vi "Fetch Waveform (Waveform Data Type)2.vi"(8 "error in (no error)":errorcluster, 9 "Maximum Time (10000ms)":u32=10000, 10 "Channel (0: Channel 1)":u16(ring) items=["Channel 1", "Channel 2", "Channel 3", "Channel 4", "Math", "Reference 1", "Reference 2", "Reference 3", "Reference 4", "D0", "D1", "D2", "D3", "D4", "D5", "D6", "D7", "D8", "D9", "D10", "D11", "D12", "D13", "D14", "D15", "Amplitude", "Frequency", "Phase", "Normal", "Average", "Maximum Peak Hold", "Minimum Peak Hold"], 11 "VISA resource name":refnum<visa-resource-name>) -> (0 "error out":errorcluster, 2 "Waveform Data":waveform(dbl)(graph), 3 "VISA resource name out":refnum<visa-resource-name>)   [LabVIEW 2011]
doc: "Returns the waveform that an oscilloscope acquires for a channel you specify. An acquisition that you initiate before calling this VI generates the waveform.\n\nYou first enable channels with the Configure Channel VI. Then you use the Initiate VI to start an acquisition on the enabled channels. An oscilloscope concurrently acquires waveforms for these channels. You must call the Fetch Waveform VI separately to obtain waveforms for each enabled channel.\nHowever, you also can call the Read Waveform VI instead of using the above low-level VIs.\n\n<B>Note</B>: Use the Fetch Waveform VI only with other low-level VIs, such as the Initiate VI, the Abort VI, and the Fetch Waveform Measurement VI. High-level VIs, such as the Read Waveform VI, automatically incorporate the functions of the Initiate VI and the Fetch Waveform VI. The Fetch Waveform VI does not check the status of an instrument."
uses:
  <instrlib>/Tektronix DPO MSO 2000 4000 Series/Tektronix DPO MSO 2000 4000 Series.lvlib
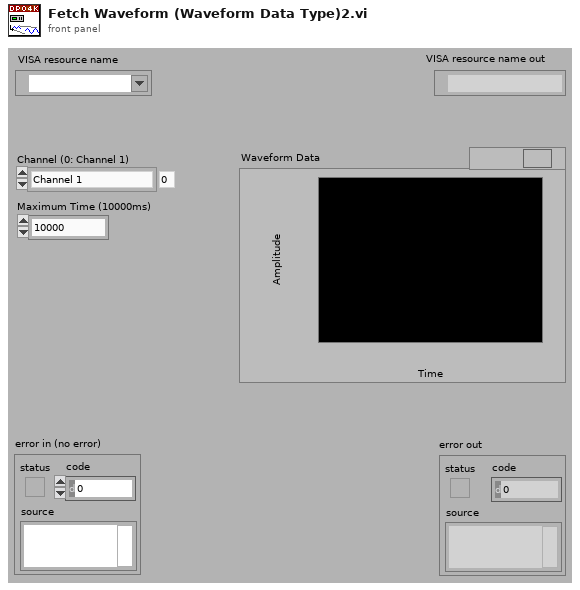
[diagram p1: front panel]
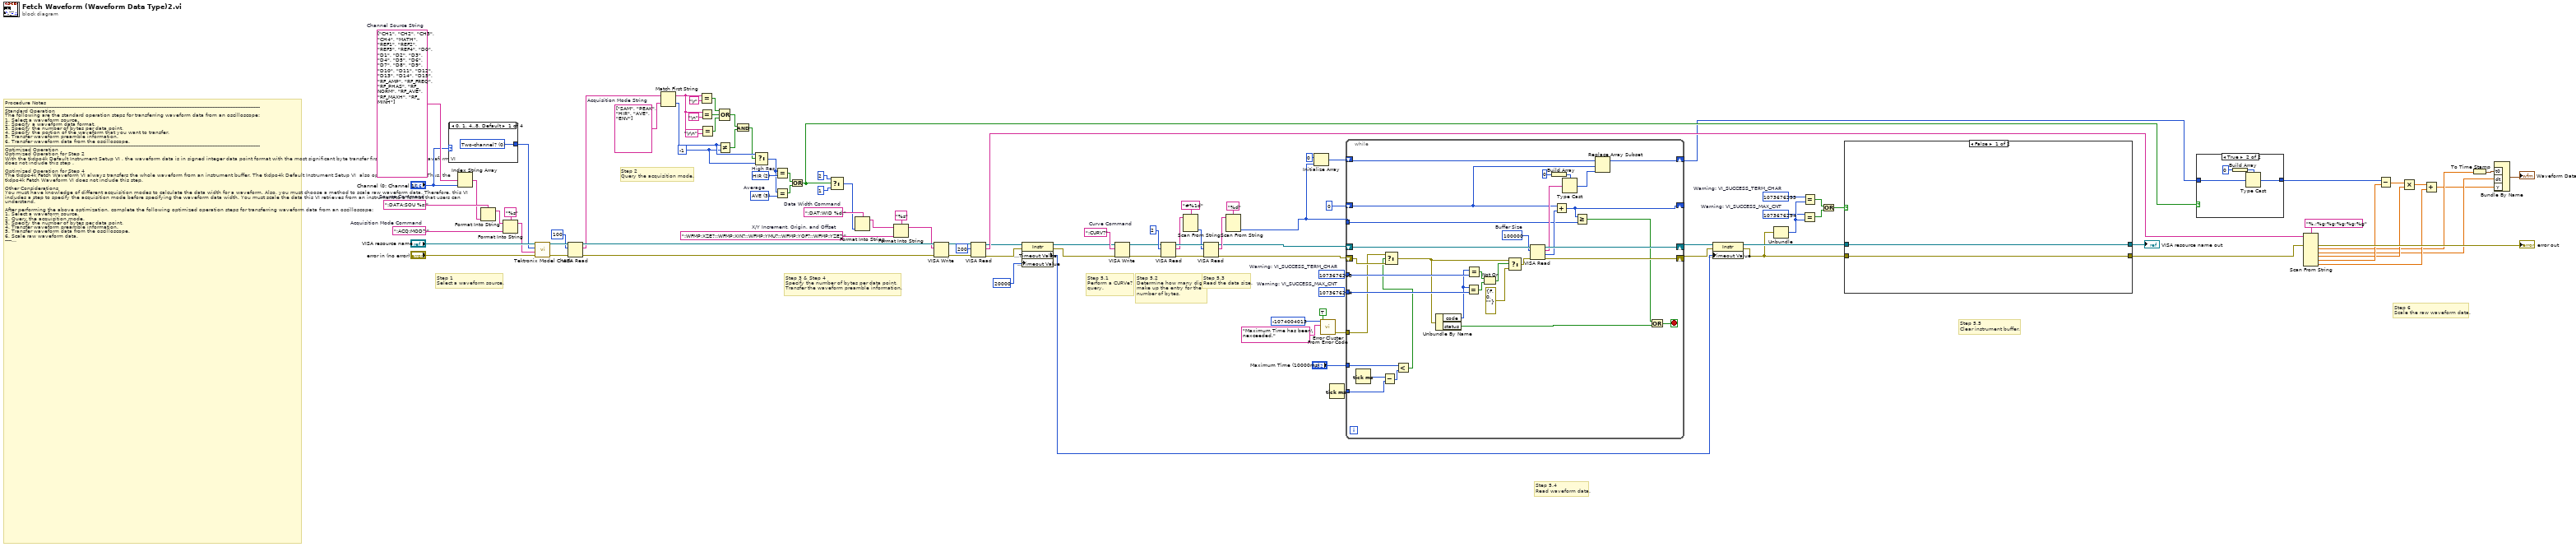
[diagram p0: block diagram]
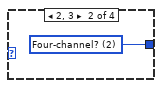
[diagram p2: hidden frame]
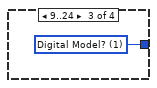
[diagram p3: hidden frame]
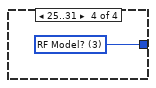
[diagram p4: hidden frame]
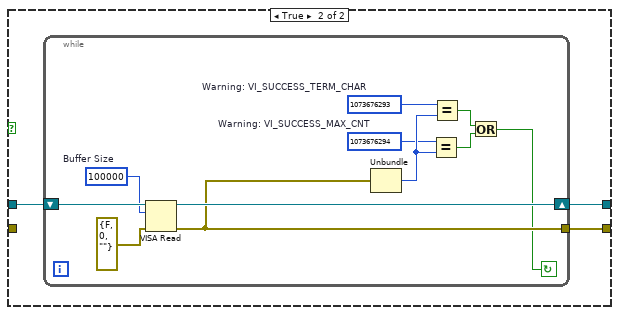
[diagram p6: hidden frame]
diagram:
  w44 = 1073676294  # Warning: VI_SUCCESS_MAX_CNT
  w45 = 1073676293  # Warning: VI_SUCCESS_TERM_CHAR
  w48 = 1073676294  # Warning: VI_SUCCESS_MAX_CNT
  w47 = 1073676293  # Warning: VI_SUCCESS_TERM_CHAR
  w57 = -1 ("y")
  w84 = ":CURV?"  # Curve Command
  w94 = ":DAT:WID %d;"  # Data Width Command
  w99 = u16 3 items=["SAM", "PEAK", "HIR", "AVE", "ENV"]  # Average
  w100 = u16 2 items=["SAM", "PEAK", "HIR", "AVE", "ENV"]  # High Res
  w69 = string[] ["SAM", "PEAK", "HIR", "AVE", "ENV"]  # Acquisition Mode String
  w93 = ":ACQ:MOD?;"  # Acquisition Mode Command
  w105 = string[] ["CH1", "CH2", "CH3", "CH4", "MATH", "REF1", "REF2", "REF3", "REF4", "D0", "D1", "D2", "D3", "D4", "D5", "D6", "D7", "D8", "D9", "D10", "D11", "D12", "D13", "D14", "D15", "RF_AMP", "RF_FREQ", "RF_PHAS", "RF_NORM", "RF_AVE", "RF_MAXH", "RF_MINH"]  # Channel Source String
  w104 = ":DATA:SOU %s;"  # Source Command
  w91 = ":WFMP:XZE?;:WFMP:XIN?;:WFMP:YMU?;:WFMP:YOF?;:WFMP:YZE?;"  # X/Y Increment, Origin, and Offset
  # "Step 6    \nScale the raw waveform data."
  # "Step 5.5    \nClear instrument buffer."
  # "Step 5.4   \nRead waveform data."
  # "Step 5.3      \nRead the data size."
  # "Step 5.2      \nDetermine how many digits\nmake up the entry for the \nnumber of bytes."
  # "Step 5.1      \nPerform a CURVe?\nquery."
  # "Step 3 & Step 4         \nSpecify the number of bytes per data point.\nTransfer the waveform preamble information."
  # "Step 2        \nQuery the acquisition mode."
  # "Step 1 \nSelect a waveform source."
  # "Procedure Notes\n-----------------------------------------------------------------------------------------------------------------------------------------------------------\nStandard Operation\nThe following are the standard operation steps for transferring waveform data from an oscilloscope:\n1. Select a waveform source.\n2. Specify a waveform data format.\n3. Specify the number of bytes per data point.\n4. Specify the portion of the waveform that you want to transfer.\n5. Transfer waveform preamble information.\n6. Transfer waveform data from the oscilloscope.\n-----------------------------------------------------------------------------------------------------------------------------------------------------------\nOptimized Operation\nOptimized Operation for Step 2\nWith the tkdpo4k Default Instrument Setup VI , the waveform data is in signed integer data point format with the most significant byte transfer first. Thus, the Fetch Waveform VI does not include this step . \n\nOptimized Operation for Step 4 \nThe tkdpo4k Fetch Waveform VI always transfers the whole waveform from an instrument buffer. The tkdpo4k Default Instrument Setup VI  also operates in this way. Thus, the tkdpo4k Fetch Waveform VI does not include this step. \n\nOther Considerations\nYou must have knowledge of different acquisition modes to calculate the data width for a waveform. Also, you must choose a method to scale raw waveform data. Therefore, this VI includes a step to specify the acquisition mode before specifying the waveform data width. You must scale the data this VI retrieves from an instrument to a format that users can understand.\n\nAfter performing the above optimization, complete the following optimized operation steps for transferring waveform data from an oscilloscope:\n1. Select a waveform source.\n2. Query the acquisition mode.\n3. Specify the number of bytes per data point.\n4. Transfer waveform preamble information.\n5. Transfer waveform data from the oscilloscope.\n6. Scale raw waveform data.\n-----------------------------------------------------------------------------------------------------------------------------------------------------------\nDetailed Steps\nThe following steps detail the behavior of this VI:\n1. Select a waveform source. \n2. Query and determine the acquisition mode. A correct determination is critical to steps 3 and 6.\n    -----------------------------------------------\n    Acquisition Mode |  Data Width   \n    -----------------------------------------------\n    Normal                       |   1                      \n    -----------------------------------------------\n    Peak Detect               |   1                      \n    -----------------------------------------------\n    Hi Res                        |   2                      \n    -----------------------------------------------\n    Envelope                   |   1                      \n    ----------------------------------------------- \n    Average                    |   2                      \n    -----------------------------------------------\n3. Specify the number of bytes per data point. For the Hi Res or Average acquisition modes, set the data width to 2. For all other acquisition modes, set the data width to 1.\n4. Transfer the waveform preamble information. Necessary preamble information includes XZero, XIncrement, YMultiplier, YOffset, and YZero. This VI uses XZero and XIncrement to configure the x-axis of output waveforms and uses YMultiplier, YOffset, and YZero to scale data values. This VI then parses the return string of the preamble query in step 6.\n5. Transfer waveform data from the oscilloscope.\n    5.1 Perform a CURVe? query.\n    5.2 Determine how many digits make up the entry for the number of bytes.\n    5.3 Read the data size.\n    5.4 Call the VISA Read VI repeatedly with a buffer size of 10000 until you obtain as much data as the data size specifies. Use      an 8-bit array to store the raw waveform data you obtain. \n    5.5 Continue reading the data remaining in the instrument buffer until the buffer is empty.\n6. Scale the raw waveform data.\n    6.1 Cast the waveform data to a 16-bit array if the data width is 2 . Split the waveform data into a minimum and a maximum data array if the acquisition mode is Peak Detect or Envelope. This VI skips this step if the data width is 1.\n    6.2 Parse the preamble information.\n    6.3 Scale the waveform data according to the following formula:\n          Data_Value_in_units = (Raw_Data_Value - YOffset) * YMultiplier + YZero\n          The resulting waveform data has a unit of volts.\n    6.4 Build a waveform graph."
  n1 = case shown="0, 1, 4..8, Default" "Channel (0: Channel 1)" {
    tunnel: [w106 w107 w108 w109] -> w1
    frame 0, 1, 4..8, Default {
      w106 = u16 0 items=["Two-channel?", "Digital Model?", "Four-channel?", "RF Model?"] ("Oscilloscope Model Tests (3: RF Model?)")
    }
    frame 2, 3 {
      w107 = u16 2 items=["Two-channel?", "Digital Model?", "Four-channel?", "RF Model?"] ("Oscilloscope Model Tests (3: RF Model?)")
    }
    frame 9..24 {
      w108 = u16 1 items=["Two-channel?", "Digital Model?", "Four-channel?", "RF Model?"] ("Oscilloscope Model Tests (3: RF Model?)")
    }
    frame 25..31 {
      w109 = u16 3 items=["Two-channel?", "Digital Model?", "Four-channel?", "RF Model?"] ("Oscilloscope Model Tests (3: RF Model?)")
    }
  }
  n2 = Index String Array(1:"Channel (0: Channel 1)", 2:w105) -> (0:w103:string)  [unwired: 1 in]
  n3 = Format Into String(format string=w104, w103) -> (resulting string=w102:string)  [unwired: 2 in, 1 out]
  n4 = Format Into String(format string="%s", initial string=w102, w93) -> (resulting string=w6:string)  [unwired: 1 in, 1 out]
  n5 = call <instrlib>:"Tektronix Model Check.vi"("error in (no error)"="error in (no error)", "Command String"=w6, "Oscilloscope Model Tests (3: RF Model?)"=w1, "VISA resource name"="VISA resource name") -> ("error out"=w4:errorcluster, "VISA resource name out"=w5:refnum<visa-resource-name>)  [unwired: 6 in]
  n6 = VISA Read(VISA resource name=w5, byte count=u32 100, error in (no error)=w4) -> (VISA resource name out=w90:refnum<visa-resource-name>, read buffer=w68:string, error out=w89:errorcluster)  [unwired: 1 out]
  n7 = Match First String(2:w69, 3:w68) -> (0:w58:i32, 1:w64:string)
  n8 = Equal?(x=w64, y="\r") -> (x = y?=w63:bool)
  n9 = Equal?(x=w64, y="\n") -> (x = y?=w62:bool)
  n10 = Equal?(x=w64, y="\r\n") -> (x = y?=w61:bool)
  n11 = Not Equal?(x=w58, y=w57) -> (x != y?=w59:bool)
  n12 = Compound Arithmetic op=OR(w63, w62, w61) -> (w60:bool)
  n13 = And(x=w60, y=w59) -> (x .and. y?=w56:bool)
  n14 = Select(t=w58, s=w56, f=w57) -> (s? t:f=w43:i32)
  n15 = Equal?(x=w43, y=w100) -> (x = y?=w98:bool)
  n16 = Equal?(x=w43, y=w99) -> (x = y?=w97:bool)
  n17 = Or(x=w98, y=w97) -> (x .or. y?=w42:bool)
  n18 = Select(t=2 ("f"), s=w42, f=1) -> (s? t:f=w74:i32)
  n19 = Format Into String(format string=w94, w74) -> (resulting string=w88:string)  [unwired: 2 in, 1 out]
  n20 = Format Into String(format string="%s", initial string=w88, w91) -> (resulting string=w75:string)  [unwired: 1 in, 1 out]
  n21 = VISA Write(VISA resource name=w90, write buffer=w75, error in (no error)=w89) -> (VISA resource name out=w86:refnum<visa-resource-name>, error out=w85:errorcluster)  [unwired: 1 out]
  n22 = VISA Read(VISA resource name=w86, byte count=u32 200, error in (no error)=w85) -> (VISA resource name out=w16:refnum<visa-resource-name>, read buffer=w73:string, error out=w15:errorcluster)  [unwired: 1 out]
  n23 = property class="Instr"(reference=w16, error in=w15, "General Settings:Timeout Value"=u32 20000) -> (reference out=w14:refnum<visa-resource-name>, error out=w12:errorcluster, "General Settings:Timeout Value"=w25:u32)
  n24 = VISA Write(VISA resource name=w14, write buffer=w84, error in (no error)=w12) -> (VISA resource name out=w13:refnum<visa-resource-name>, error out=w11:errorcluster)  [unwired: 1 out]
  n25 = VISA Read(VISA resource name=w13, byte count=u32 2, error in (no error)=w11) -> (VISA resource name out=w81:refnum<visa-resource-name>, read buffer=w79:string, error out=w80:errorcluster)  [unwired: 1 out]
  n26 = Scan From String(format string="#%1d", input string=w79) -> (output 1=w78:i32)  [unwired: 3 in, 3 out]
  n27 = VISA Read(VISA resource name=w81, byte count=w78, error in (no error)=w80) -> (VISA resource name out=w10:refnum<visa-resource-name>, read buffer=w76:string, error out=w9:errorcluster)  [unwired: 1 out]
  n28 = Scan From String(format string="%d", input string=w76) -> (output 1=w55:i32)  [unwired: 3 in, 3 out]
  n29 = Initialize Array(i8 0 ("element"), w55) -> (w53:i8[])
  n30 = call <vilib>:"Error Cluster From Error Code.vi"("show call chain? (False)"=TRUE, "error message (\"\")"="Maximum Time has been\nexceeded." ("error message (\"\")"), "error code (0)"=-1074004013) -> ("error out"=w17:errorcluster)  [unwired: 6 in]
  n31 = Tick Count (ms)() -> (millisecond timer value=w22:u32)
  n32 = while {
    shift-right: [w140] -> w27
    shift-left: w10 -> [w142]
    shift-right: [w139] -> w26
    shift-left: w9 -> [w112]
    shift-right: [w135] -> w41
    shift-left: w53 -> [w136]
    tunnel: w55 -> [w132]
    shift-right: [w129] -> _
    shift-left: 0 -> [w130]
    tunnel: w45 -> [w123]
    tunnel: w44 -> [w122]
    tunnel: w22 -> [w116]
    tunnel: "Maximum Time (10000ms)" -> [w114]
    tunnel: w17 -> [w111]
    stop <- w128 stop-if-true
    w141 = 100000  # Buffer Size
    n33 = Tick Count (ms)() -> (millisecond timer value=w117:u32)
    n34 = Subtract(x=w117, y=w116) -> (x-y=w115:u32)
    n35 = Less?(x=w114, y=w115) -> (x < y?=w110:bool)
    n36 = Select(t=w111, s=w110, f=w112) -> (s? t:f=w113:errorcluster)
    n37 = Unbundle By Name(w113) -> ("code"=w121:i32, "status"=w125:bool)
    n38 = Equal?(x=w121, y=w122) -> (x = y?=w119:bool)
    n39 = Equal?(x=w121, y=w123) -> (x = y?=w120:bool)
    n40 = Not Or(1:w119, 2:w120) -> (0:w118:bool)
    n41 = Select(t=w113, s=w118, f=errorcluster {"status"=FALSE, "code"=0, "source"=""} ("error in (no error)")) -> (s? t:f=w124:errorcluster)
    n42 = VISA Read(VISA resource name=w142, byte count=w141, error in (no error)=w124) -> (VISA resource name out=w140:refnum<visa-resource-name>, read buffer=w134:string, return count=w133:u32, error out=w139:errorcluster)
    n43 = Build Array(i8 0) -> (w138:i8[])
    n44 = Add(x=w130, y=w133) -> (x+y=w129:u32)
    n45 = Type Cast(type=w138, x=w134) -> (*(type *) &x=w131:i8[])
    n46 = Greater Or Equal?(x=w129, y=w132) -> (x >= y?=w127:bool)
    n47 = Replace Array Subset(array=w136, new element=w131, index=w130) -> (w135:i8[])
    n48 = Compound Arithmetic op=OR(w127, w125) -> (w128:bool)
  }
  n49 = property class="Instr"(reference=w27, error in=w26, "General Settings:Timeout Value"=w25) -> (reference out=w24:refnum<visa-resource-name>, error out=w23:errorcluster)
  n50 = Unbundle(w23) -> ("code"=w49:i32)  [unwired: 2 out]
  n51 = Equal?(x=w48, y=w49) -> (x = y?=w51:bool)
  n52 = Equal?(x=w47, y=w49) -> (x = y?=w52:bool)
  n53 = Or(x=w52, y=w51) -> (x .or. y?=w50:bool)
  n54 = case shown="False" w50 {
    tunnel: w24 -> [w144 w147]
    tunnel: w23 -> [w143 _]
    tunnel: [w144 w146] -> w70
    tunnel: [w143 w145] -> w72
    frame False {
    }
    frame True {
      n55 = while {
        shift-right: [w157] -> w146
        shift-left: w147 -> [w158]
        tunnel: [w150] -> w145
        stop <- w149 continue-if-true
        w152 = 1073676294  # Warning: VI_SUCCESS_MAX_CNT
        w151 = 1073676293  # Warning: VI_SUCCESS_TERM_CHAR
        w156 = u32 100000  # Buffer Size
        n56 = VISA Read(VISA resource name=w158, byte count=w156, error in (no error)=errorcluster {"status"=FALSE, "code"=0, "source"=""}) -> (VISA resource name out=w157:refnum<visa-resource-name>, error out=w150:errorcluster)  [unwired: 2 out]
        n57 = Unbundle(w150) -> ("code"=w153:i32)  [unwired: 2 out]
        n58 = Equal?(x=w152, y=w153) -> (x = y?=w154:bool)
        n59 = Equal?(x=w151, y=w153) -> (x = y?=w155:bool)
        n60 = Or(x=w155, y=w154) -> (x .or. y?=w149:bool)
      }
    }
  }
  "VISA resource name out" <- w70
  n61 = case shown="True" w42 {
    tunnel: w41 -> [w159 w161]
    tunnel: [w159 w160] -> w30
    frame False {
    }
    frame True {
      n62 = Build Array(i16 0 ("element")) -> (w162:i16[])
      n63 = Type Cast(type=w162, x=w161) -> (*(type *) &x=w160:i16[])
    }
  }
  n64 = Scan From String(format string="%.;%g;%g;%g;%g;%g", input string=w73, error in=w72) -> (error out=→"error out":errorcluster, output 1=w34:dbl, output 2=w33:dbl, output 3=w35:dbl, output 4=w36:dbl, output 5=w37:dbl)  [unwired: 6 in, 2 out]
  n65 = Subtract(x=w30, y=w36) -> (x-y=w39:dbl[])
  n66 = Multiply(x=w39, y=w35) -> (x*y=w38:dbl[])
  n67 = Add(x=w38, y=w37) -> (x+y=w32:dbl[])
  n68 = To Time Stamp(1:w34) -> (0:w31:timestamp)
  n69 = Bundle By Name("t0"=w31, "dt"=w33, "Y"=w32) -> (→"Waveform Data":waveform(dbl))  [unwired: 1 in]
